vi "ReadQualisysFile.vi"(4 "sortie d'erreur":errorcluster caption="entrée d'erreur", 6 "QualisysDataType":enum16{"6DOF", "3DTracking", "6DOF + 3D"}(ring), 7 "FichierQualisys":path=path "D:/Mesures/rururu/MeasQualisys/TestValise0017.tsv") -> (0 "error out":errorcluster, 3 "QualisysWaveforms":waveform(dbl)[](graph))   [LabVIEW 2017]
uses:
  <vilib>/Utility/miscctls.llb/LVDateTimeRec.ctl
panel:
  out "NbFrames 2":u32
  out "NbCameras 2":u32
  out "NbMarkers":u32
  out "horodatage 2":timestamp=timestamp(3568107998 s since 1904-01-01)
  out "Noms des Markers":string[](array[string])
  out "Noms des colonnes 2":string[](array[string])
  out "Freq 2":u32
  out "dt 2":dbl
  out "dt":dbl
  out "Freq":u32
  out "Noms des colonnes":string[](array[string])
  out "Noms des bodies":string[](array[string])
  out "horodatage":timestamp=timestamp(3568107998 s since 1904-01-01)
  out "NbBodies":u32
  out "NbCameras":u32
  out "NbFrames":u32
  # "6DOF indicators"
  # "3D Data indicators"
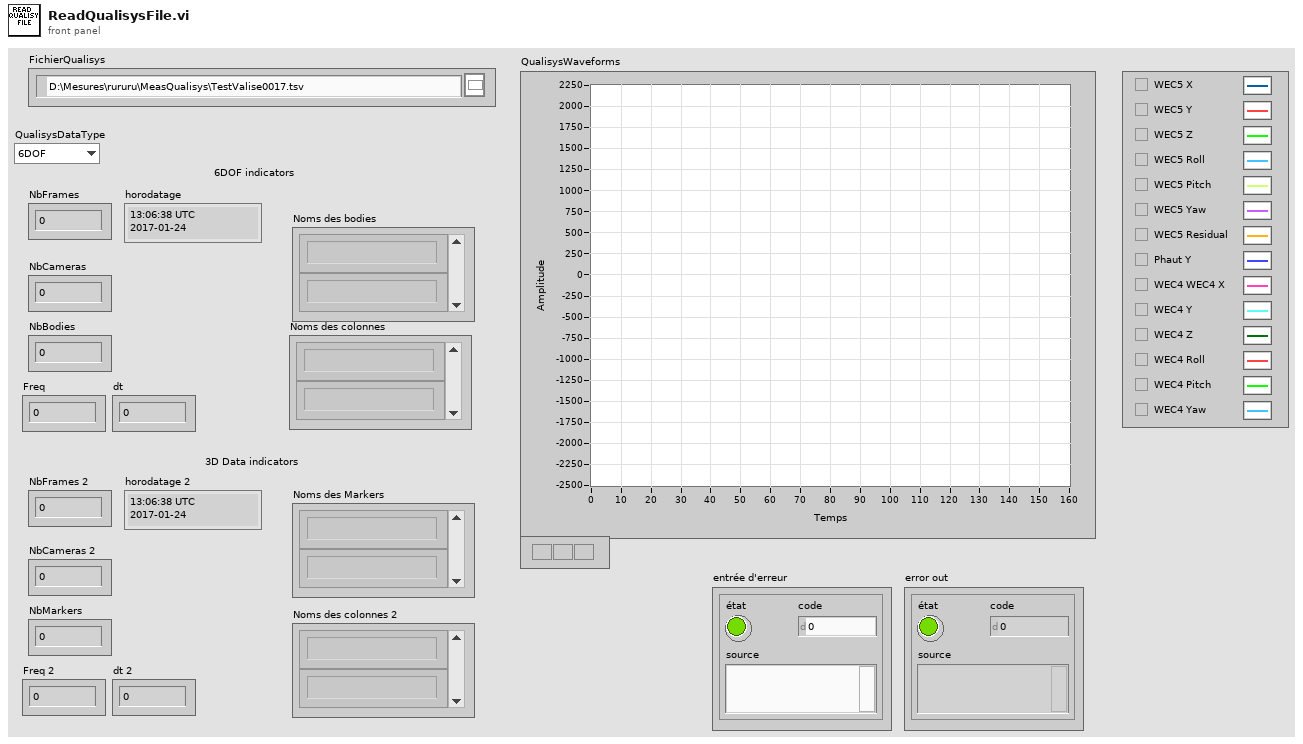
[diagram p1: front panel]
types:
  T1 = typedef "LVDateTimeRec.ctl" = cluster{"fractional second":dbl, "second":i32, "minute":i32, "hour":i32, "day of month":i32, "month":i32, "year":i32, "day of week":i32, "day of year":i32, "DST":i32}
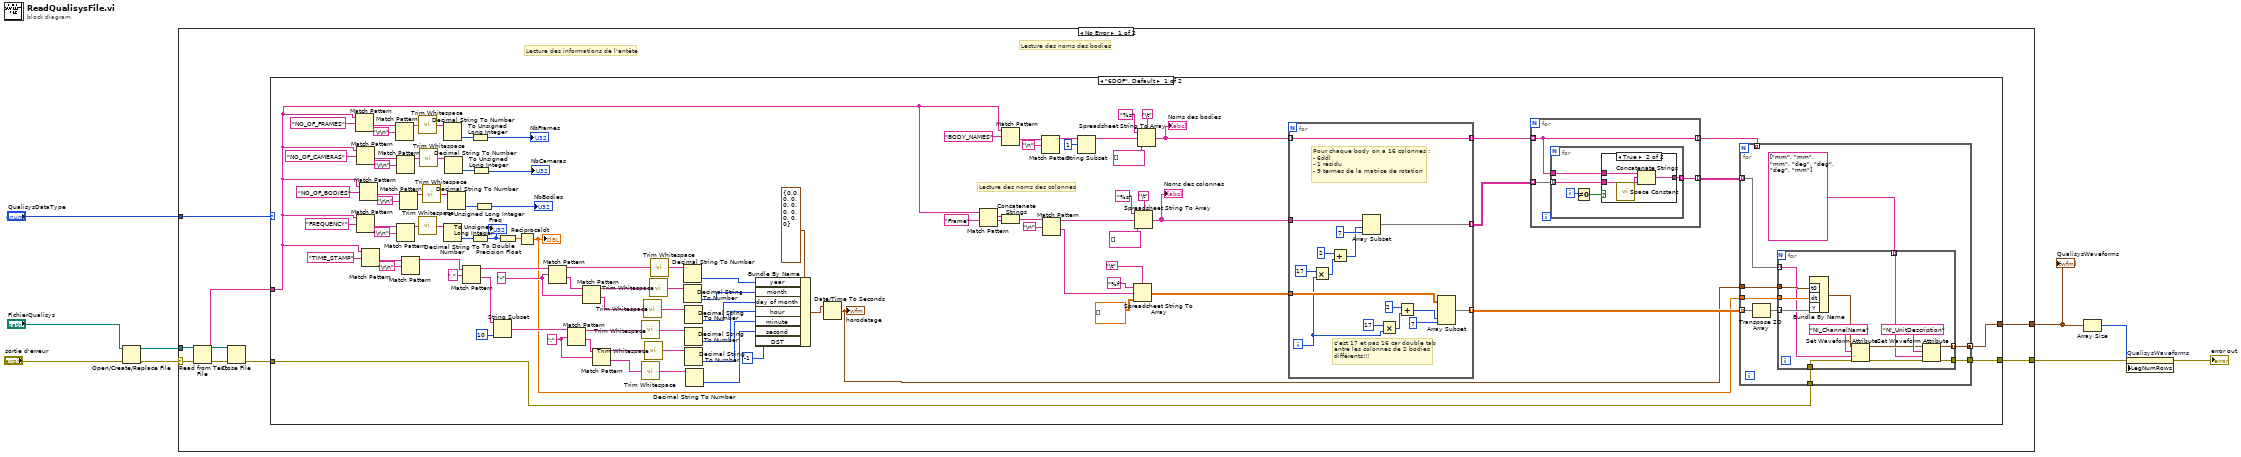
[diagram p0: block diagram]
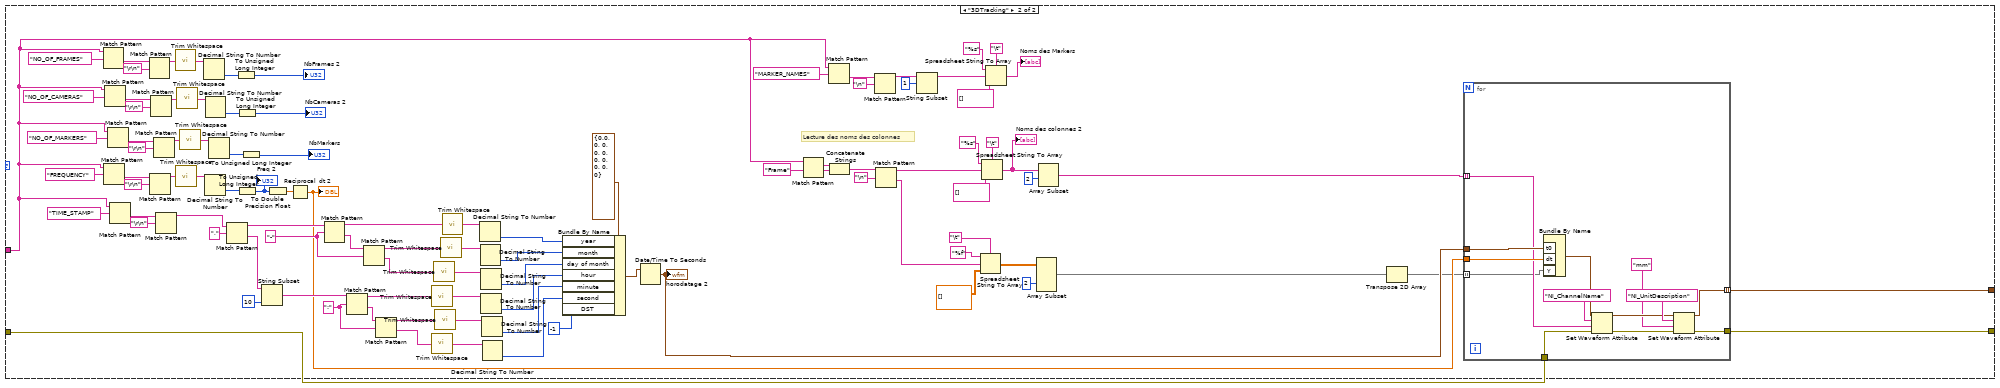
[diagram p3: hidden frame]
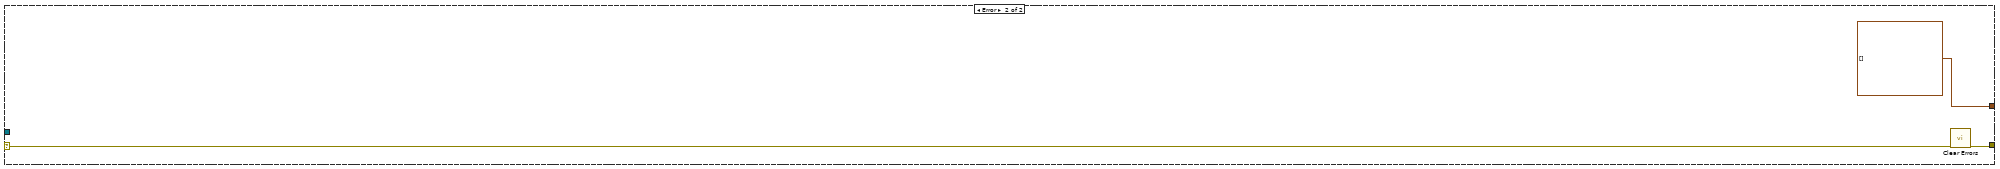
[diagram p4: hidden frame]
diagram:
  n1 = Open/Create/Replace File(file path (use dialog)="FichierQualisys", error in="sortie d'erreur") -> (refnum out=w6:refnum<file>, error out=w9:errorcluster)  [unwired: 4 in, 1 out]
  n2 = case shown="No Error" w9 {
    selector: w9 -> [w16 w281]
    tunnel: w6 -> [w15 _]
    tunnel: [w12 w282] -> w4
    tunnel: [w11 waveform(dbl)[] []] -> w5
    tunnel: "QualisysDataType" -> [w10 _]
    frame No Error {
      # "Lecture des noms des bodies"
      # "Lecture des informations de l'entête"
      n3 = Read from Text File(file (use dialog)=w15, error in=w16) -> (refnum out=w17:refnum<file>, text=w14:string, error out=w18:errorcluster)  [unwired: 2 in, 1 out]
      n4 = Close File(refnum=w17, error in=w18) -> (error out=w13:errorcluster)  [unwired: 1 out]
      n5 = case shown="\"6DOF\", Default" w10 {
        tunnel: w14 -> [w30 w185]
        tunnel: w13 -> [w22 w180]
        tunnel: [w21 w179] -> w12
        tunnel: [w20 w170] -> w11
        frame "6DOF", Default {
          w77 = ":" ("expression régulière")
          w87 = "-" ("expression régulière")
          # "Lecture des noms des colonnes"
          n6 = Match Pattern(string=w30, regular expression="NO_OF_FRAMES" ("expression régulière")) -> (after substring=w115:string)  [unwired: 1 in, 3 out]
          n7 = Match Pattern(string=w30, regular expression="FREQUENCY" ("expression régulière")) -> (after substring=w33:string)  [unwired: 1 in, 3 out]
          n8 = Match Pattern(string=w30, regular expression="NO_OF_CAMERAS" ("expression régulière")) -> (after substring=w107:string)  [unwired: 1 in, 3 out]
          n9 = Match Pattern(string=w30, regular expression="NO_OF_BODIES" ("expression régulière")) -> (after substring=w102:string)  [unwired: 1 in, 3 out]
          n10 = Match Pattern(string=w30, regular expression="TIME_STAMP" ("expression régulière")) -> (after substring=w98:string)  [unwired: 1 in, 3 out]
          n11 = Match Pattern(string=w115, regular expression="\r\n") -> (before substring=w112:string)  [unwired: 1 in, 3 out]
          n12 = Match Pattern(string=w33, regular expression="\r\n") -> (before substring=w35:string)  [unwired: 1 in, 3 out]
          n13 = Match Pattern(string=w107, regular expression="\r\n") -> (before substring=w109:string)  [unwired: 1 in, 3 out]
          n14 = Match Pattern(string=w102, regular expression="\r\n") -> (before substring=w100:string)  [unwired: 1 in, 3 out]
          n15 = Match Pattern(string=w98, regular expression="\r\n") -> (before substring=w94:string)  [unwired: 1 in, 3 out]
          n16 = call <vilib>:"Trim Whitespace.vi"("string"=w112) -> ("trimmed string"=w111:string)  [unwired: 1 in]
          n17 = call <vilib>:"Trim Whitespace.vi"("string"=w35) -> ("trimmed string"=w36:string)  [unwired: 1 in]
          n18 = call <vilib>:"Trim Whitespace.vi"("string"=w109) -> ("trimmed string"=w110:string)  [unwired: 1 in]
          n19 = call <vilib>:"Trim Whitespace.vi"("string"=w100) -> ("trimmed string"=w99:string)  [unwired: 1 in]
          n20 = Decimal String To Number(string=w111) -> (number=w114:i32)  [unwired: 2 in, 1 out]
          n21 = Decimal String To Number(string=w36) -> (number=w34:i32)  [unwired: 2 in, 1 out]
          n22 = Decimal String To Number(string=w110) -> (number=w108:i32)  [unwired: 2 in, 1 out]
          n23 = Decimal String To Number(string=w99) -> (number=w101:i32)  [unwired: 2 in, 1 out]
          n24 = Match Pattern(string=w94, regular expression="," ("expression régulière")) -> (before substring=w89:string, after substring=w75:string)  [unwired: 1 in, 2 out]
          n25 = To Unsigned Long Integer(number=w114) -> (unsigned 32bit integer=→"NbFrames":u32)
          n26 = To Unsigned Long Integer(number=w34) -> (unsigned 32bit integer=w26:u32)
          "Freq" <- w26
          n27 = To Unsigned Long Integer(number=w108) -> (unsigned 32bit integer=→"NbCameras":u32)
          n28 = To Unsigned Long Integer(number=w101) -> (unsigned 32bit integer=→"NbBodies":u32)
          n29 = String Subset(string=w75, length (rest)=10 ("longueur (reste)")) -> (substring=w74:string)  [unwired: 1 in]
          n30 = To Double Precision Float(number=w26) -> (double precision float=w25:dbl)
          n31 = Reciprocal(x=w25) -> (1/x=w24:dbl)
          "dt" <- w24
          n32 = Match Pattern(string=w89, regular expression=w87) -> (before substring=w86:string, after substring=w88:string)  [unwired: 1 in, 2 out]
          n33 = Match Pattern(string=w74, regular expression=w77) -> (before substring=w78:string, after substring=w76:string)  [unwired: 1 in, 2 out]
          n34 = Match Pattern(string=w88, regular expression=w87) -> (before substring=w84:string, after substring=w83:string)  [unwired: 1 in, 2 out]
          n35 = Match Pattern(string=w76, regular expression=w77) -> (before substring=w79:string, after substring=w80:string)  [unwired: 1 in, 2 out]
          n36 = call <vilib>:"Trim Whitespace.vi"("string"=w78) -> ("trimmed string"=w66:string)  [unwired: 1 in]
          n37 = call <vilib>:"Trim Whitespace.vi"("string"=w80) -> ("trimmed string"=w64:string)  [unwired: 1 in]
          n38 = call <vilib>:"Trim Whitespace.vi"("string"=w83) -> ("trimmed string"=w67:string)  [unwired: 1 in]
          n39 = call <vilib>:"Trim Whitespace.vi"("string"=w79) -> ("trimmed string"=w65:string)  [unwired: 1 in]
          n40 = call <vilib>:"Trim Whitespace.vi"("string"=w84) -> ("trimmed string"=w68:string)  [unwired: 1 in]
          n41 = call <vilib>:"Trim Whitespace.vi"("string"=w86) -> ("trimmed string"=w69:string)  [unwired: 1 in]
          n42 = Decimal String To Number(string=w69) -> (number=w85:i32)  [unwired: 2 in, 1 out]
          n43 = Decimal String To Number(string=w68) -> (number=w82:i32)  [unwired: 2 in, 1 out]
          n44 = Decimal String To Number(string=w67) -> (number=w81:i32)  [unwired: 2 in, 1 out]
          n45 = Decimal String To Number(string=w66) -> (number=w72:i32)  [unwired: 2 in, 1 out]
          n46 = Decimal String To Number(string=w65) -> (number=w71:i32)  [unwired: 2 in, 1 out]
          n47 = Decimal String To Number(string=w64) -> (number=w70:i32)  [unwired: 2 in, 1 out]
          n48 = Bundle By Name(cluster=T1 {"fractional second"=0.0, "second"=0, "minute"=0, "hour"=0, "day of month"=0, "month"=0, "year"=0, "day of week"=0, "day of year"=0, "DST"=0} ("cluster date/heure"), "year"=w85, "month"=w82, "day of month"=w81, "hour"=w72, "minute"=w71, "second"=w70, "DST"=-1) -> (w92:T1)
          n49 = Date/Time To Seconds(2:w92) -> (0:w23:timestamp)  [unwired: 1 in]
          "horodatage" <- w23
          n50 = Match Pattern(string=w30, regular expression="Frame" ("expression régulière")) -> (match substring=w49:string, after substring=w48:string)  [unwired: 1 in, 2 out]
          n51 = Match Pattern(string=w30, regular expression="BODY_NAMES" ("expression régulière")) -> (after substring=w63:string)  [unwired: 1 in, 3 out]
          n52 = Concatenate Strings(w49, w48) -> (w47:string)
          n53 = Match Pattern(string=w63, regular expression="\n") -> (before substring=w60:string)  [unwired: 1 in, 3 out]
          n54 = Match Pattern(string=w47, regular expression="\n") -> (before substring=w46:string, after substring=w45:string)  [unwired: 1 in, 2 out]
          n55 = String Subset(string=w60, offset (0)=1) -> (substring=w56:string)  [unwired: 1 in]
          n56 = Spreadsheet String To Array(delimiter (Tab)="\t", format string="%f" ("chaîne de format"), spreadsheet string=w45, array type (2D Dbl)=dbl[][] [] ("type de tableau (2D de dbl)")) -> (array=w39:dbl[][])
          n57 = Spreadsheet String To Array(delimiter (Tab)="\t", format string="%s" ("chaîne de format"), spreadsheet string=w46, array type (2D Dbl)=string[] [] ("type de tableau (2D de dbl)")) -> (array=w40:string[])
          "Noms des colonnes" <- w40
          n58 = Spreadsheet String To Array(delimiter (Tab)="\t", format string="%s" ("chaîne de format"), spreadsheet string=w56, array type (2D Dbl)=string[] [] ("type de tableau (2D de dbl)")) -> (array=w41:string[])
          "Noms des bodies" <- w41
          n59 = for {
            tunnel: w40 -> [w158]
            tunnel: w41 -> [w153] mode=indexing
            tunnel: [w157] -> w38 mode=indexing
            tunnel: w39 -> [w156]
            tunnel: [w154] -> w27 mode=indexing
            tunnel: [w153] -> w37 mode=indexing
            i -> [w155]
            # "Pour chaque body on a 16 colonnes :\n- 6ddl\n- 1 résidu\n- 9 termes de la matrice de rotation"
            # "c'est 17 et pas 16 car double tab\nentre les colonnes de 2 bodies\ndifférents!!!"
            n60 = Multiply(x=17 ("indice"), y=w155) -> (x*y=w166:i32)
            n61 = Add(x=2 ("indice"), y=w166) -> (x+y=w163:i32)
            n62 = Array Subset(array=w158, index=w163, length=7 ("longueur")) -> (w157:string[])
            n63 = Multiply(x=17 ("indice"), y=w155) -> (x*y=w160:i32)
            n64 = Add(x=2 ("indice"), y=w160) -> (x+y=w159:i32)
            n65 = Array Subset(array=w156, index (col)=w159, length (col)=7 ("longueur")) -> (w154:dbl[][])  [unwired: 2 in]
          }
          n66 = for {
            tunnel: w38 -> [w142] mode=indexing
            tunnel: [w141] -> w28 mode=indexing
            tunnel: w37 -> [w140] mode=indexing
            tunnel: [w140] -> w29 mode=indexing
            n67 = for {
              tunnel: w142 -> [w147] mode=indexing
              tunnel: [w146] -> w141 mode=indexing
              tunnel: w140 -> [w143]
              i -> [w145]
              n68 = Not Equal To 0?(x=w145) -> (x != 0?=w144:bool)
              n69 = case shown="True" w144 {
                tunnel: w147 -> [w148 w151]
                tunnel: [w148 w152] -> w146
                tunnel: w143 -> [_ w149]
                frame False {
                }
                frame True {
                  n70 = call <vilib>:"Space Constant.vi"() -> ("String"=w150:string)
                  n71 = Concatenate Strings(w149, w150, w151) -> (w152:string)
                }
              }
            }
          }
          n72 = for {
            tunnel: w29 -> [_] mode=indexing
            tunnel: w28 -> [w120] mode=indexing
            tunnel: w27 -> [w124] mode=indexing
            tunnel: w24 -> [w125]
            tunnel: w23 -> [w126]
            tunnel: w22 -> [w122]
            tunnel: [w121] -> w21
            tunnel: [w118] -> w20 mode=concatenating
            n73 = Transpose 2D Array(2D array=w124) -> (transposed array=w123:dbl[][])
            n74 = for {
              tunnel: w126 -> [w139]
              tunnel: w125 -> [w138]
              tunnel: w123 -> [w137] mode=indexing
              tunnel: w122 -> [w131]
              tunnel: [w130] -> w121
              tunnel: w120 -> [w129] mode=indexing
              tunnel: string[] ["mm", "mm", "mm", "deg", "deg", "deg", "mm"] -> [w128] mode=indexing
              tunnel: [w127] -> w118 mode=indexing
              n75 = Bundle By Name("t0"=w139, "dt"=w138, "Y"=w137) -> (w132:waveform(dbl))  [unwired: 1 in]
              n76 = Set Waveform Attribute(4:w131, 5:w129, 6:"NI_ChannelName" ("nom"), 7:w132) -> (0:w134:errorcluster, 3:w133:waveform(dbl))  [unwired: 1 out]
              n77 = Set Waveform Attribute(4:w134, 5:w128, 6:"NI_UnitDescription" ("nom"), 7:w133) -> (0:w130:errorcluster, 3:w127:waveform(dbl))  [unwired: 1 out]
            }
          }
        }
        frame "3DTracking" {
          w227 = ":" ("expression régulière")
          w237 = "-" ("expression régulière")
          # "Lecture des noms des colonnes"
          n78 = Match Pattern(string=w185, regular expression="NO_OF_FRAMES" ("expression régulière")) -> (after substring=w265:string)  [unwired: 1 in, 3 out]
          n79 = Match Pattern(string=w185, regular expression="FREQUENCY" ("expression régulière")) -> (after substring=w188:string)  [unwired: 1 in, 3 out]
          n80 = Match Pattern(string=w185, regular expression="NO_OF_CAMERAS" ("expression régulière")) -> (after substring=w257:string)  [unwired: 1 in, 3 out]
          n81 = Match Pattern(string=w185, regular expression="NO_OF_MARKERS" ("expression régulière")) -> (after substring=w252:string)  [unwired: 1 in, 3 out]
          n82 = Match Pattern(string=w185, regular expression="TIME_STAMP" ("expression régulière")) -> (after substring=w248:string)  [unwired: 1 in, 3 out]
          n83 = Match Pattern(string=w265, regular expression="\r\n") -> (before substring=w262:string)  [unwired: 1 in, 3 out]
          n84 = Match Pattern(string=w188, regular expression="\r\n") -> (before substring=w190:string)  [unwired: 1 in, 3 out]
          n85 = Match Pattern(string=w257, regular expression="\r\n") -> (before substring=w259:string)  [unwired: 1 in, 3 out]
          n86 = Match Pattern(string=w252, regular expression="\r\n") -> (before substring=w250:string)  [unwired: 1 in, 3 out]
          n87 = Match Pattern(string=w248, regular expression="\r\n") -> (before substring=w244:string)  [unwired: 1 in, 3 out]
          n88 = call <vilib>:"Trim Whitespace.vi"("string"=w262) -> ("trimmed string"=w261:string)  [unwired: 1 in]
          n89 = call <vilib>:"Trim Whitespace.vi"("string"=w190) -> ("trimmed string"=w191:string)  [unwired: 1 in]
          n90 = call <vilib>:"Trim Whitespace.vi"("string"=w259) -> ("trimmed string"=w260:string)  [unwired: 1 in]
          n91 = call <vilib>:"Trim Whitespace.vi"("string"=w250) -> ("trimmed string"=w249:string)  [unwired: 1 in]
          n92 = Decimal String To Number(string=w261) -> (number=w264:i32)  [unwired: 2 in, 1 out]
          n93 = Decimal String To Number(string=w191) -> (number=w189:i32)  [unwired: 2 in, 1 out]
          n94 = Decimal String To Number(string=w260) -> (number=w258:i32)  [unwired: 2 in, 1 out]
          n95 = Decimal String To Number(string=w249) -> (number=w251:i32)  [unwired: 2 in, 1 out]
          n96 = Match Pattern(string=w244, regular expression="," ("expression régulière")) -> (before substring=w239:string, after substring=w225:string)  [unwired: 1 in, 2 out]
          n97 = To Unsigned Long Integer(number=w264) -> (unsigned 32bit integer=→"NbFrames 2":u32)
          n98 = To Unsigned Long Integer(number=w189) -> (unsigned 32bit integer=w184:u32)
          "Freq 2" <- w184
          n99 = To Unsigned Long Integer(number=w258) -> (unsigned 32bit integer=→"NbCameras 2":u32)
          n100 = To Unsigned Long Integer(number=w251) -> (unsigned 32bit integer=→"NbMarkers":u32)
          n101 = String Subset(string=w225, length (rest)=10 ("longueur (reste)")) -> (substring=w224:string)  [unwired: 1 in]
          n102 = To Double Precision Float(number=w184) -> (double precision float=w183:dbl)
          n103 = Reciprocal(x=w183) -> (1/x=w182:dbl)
          "dt 2" <- w182
          n104 = Match Pattern(string=w239, regular expression=w237) -> (before substring=w236:string, after substring=w238:string)  [unwired: 1 in, 2 out]
          n105 = Match Pattern(string=w224, regular expression=w227) -> (before substring=w228:string, after substring=w226:string)  [unwired: 1 in, 2 out]
          n106 = Match Pattern(string=w238, regular expression=w237) -> (before substring=w234:string, after substring=w233:string)  [unwired: 1 in, 2 out]
          n107 = Match Pattern(string=w226, regular expression=w227) -> (before substring=w229:string, after substring=w230:string)  [unwired: 1 in, 2 out]
          n108 = call <vilib>:"Trim Whitespace.vi"("string"=w228) -> ("trimmed string"=w216:string)  [unwired: 1 in]
          n109 = call <vilib>:"Trim Whitespace.vi"("string"=w230) -> ("trimmed string"=w214:string)  [unwired: 1 in]
          n110 = call <vilib>:"Trim Whitespace.vi"("string"=w233) -> ("trimmed string"=w217:string)  [unwired: 1 in]
          n111 = call <vilib>:"Trim Whitespace.vi"("string"=w229) -> ("trimmed string"=w215:string)  [unwired: 1 in]
          n112 = call <vilib>:"Trim Whitespace.vi"("string"=w234) -> ("trimmed string"=w218:string)  [unwired: 1 in]
          n113 = call <vilib>:"Trim Whitespace.vi"("string"=w236) -> ("trimmed string"=w219:string)  [unwired: 1 in]
          n114 = Decimal String To Number(string=w219) -> (number=w235:i32)  [unwired: 2 in, 1 out]
          n115 = Decimal String To Number(string=w218) -> (number=w232:i32)  [unwired: 2 in, 1 out]
          n116 = Decimal String To Number(string=w217) -> (number=w231:i32)  [unwired: 2 in, 1 out]
          n117 = Decimal String To Number(string=w216) -> (number=w222:i32)  [unwired: 2 in, 1 out]
          n118 = Decimal String To Number(string=w215) -> (number=w221:i32)  [unwired: 2 in, 1 out]
          n119 = Decimal String To Number(string=w214) -> (number=w220:i32)  [unwired: 2 in, 1 out]
          n120 = Bundle By Name(cluster=T1 {"fractional second"=0.0, "second"=0, "minute"=0, "hour"=0, "day of month"=0, "month"=0, "year"=0, "day of week"=0, "day of year"=0, "DST"=0} ("cluster date/heure"), "year"=w235, "month"=w232, "day of month"=w231, "hour"=w222, "minute"=w221, "second"=w220, "DST"=-1) -> (w242:T1)
          n121 = Date/Time To Seconds(2:w242) -> (0:w181:timestamp)  [unwired: 1 in]
          "horodatage 2" <- w181
          n122 = Match Pattern(string=w185, regular expression="Frame" ("expression régulière")) -> (match substring=w199:string, after substring=w198:string)  [unwired: 1 in, 2 out]
          n123 = Match Pattern(string=w185, regular expression="MARKER_NAMES" ("expression régulière")) -> (after substring=w213:string)  [unwired: 1 in, 3 out]
          n124 = Concatenate Strings(w199, w198) -> (w197:string)
          n125 = Match Pattern(string=w213, regular expression="\n") -> (before substring=w210:string)  [unwired: 1 in, 3 out]
          n126 = Match Pattern(string=w197, regular expression="\n") -> (before substring=w196:string, after substring=w195:string)  [unwired: 1 in, 2 out]
          n127 = String Subset(string=w210, offset (0)=1) -> (substring=w206:string)  [unwired: 1 in]
          n128 = Spreadsheet String To Array(delimiter (Tab)="\t", format string="%f" ("chaîne de format"), spreadsheet string=w195, array type (2D Dbl)=dbl[][] [] ("type de tableau (2D de dbl)")) -> (array=w177:dbl[][])
          n129 = Spreadsheet String To Array(delimiter (Tab)="\t", format string="%s" ("chaîne de format"), spreadsheet string=w196, array type (2D Dbl)=string[] [] ("type de tableau (2D de dbl)")) -> (array=w175:string[])
          "Noms des colonnes 2" <- w175
          n130 = Spreadsheet String To Array(delimiter (Tab)="\t", format string="%s" ("chaîne de format"), spreadsheet string=w206, array type (2D Dbl)=string[] [] ("type de tableau (2D de dbl)")) -> (array=→"Noms des Markers":string[])
          n131 = Array Subset(array=w177, index (col)=2 ("index")) -> (w172:dbl[][])  [unwired: 3 in]
          n132 = Array Subset(array=w175, index=2) -> (w171:string[])  [unwired: 1 in]
          n133 = Transpose 2D Array(2D array=w172) -> (transposed array=w169:dbl[][])
          n134 = for {
            tunnel: w169 -> [w268] mode=indexing
            tunnel: w182 -> [w279]
            tunnel: w181 -> [w280]
            tunnel: w180 -> [w278]
            tunnel: [w277] -> w179
            tunnel: w171 -> [w270] mode=indexing
            tunnel: [w269] -> w170 mode=indexing
            n135 = Bundle By Name("t0"=w280, "dt"=w279, "Y"=w268) -> (w272:waveform(dbl))  [unwired: 1 in]
            n136 = Set Waveform Attribute(4:w278, 5:w270, 6:"NI_ChannelName" ("nom"), 7:w272) -> (0:w274:errorcluster, 3:w273:waveform(dbl))  [unwired: 1 out]
            n137 = Set Waveform Attribute(4:w274, 5:"mm" ("expression régulière"), 6:"NI_UnitDescription" ("nom"), 7:w273) -> (0:w277:errorcluster, 3:w269:waveform(dbl))  [unwired: 1 out]
          }
        }
      }
    }
    frame Error {
      n138 = call <vilib>:"Clear Errors.vi"("error in (no error)"=w281) -> ("error out"=w282:errorcluster)  [unwired: 5 in, 1 out]
    }
  }
  "QualisysWaveforms" <- w5
  n139 = Array Size(array=w5) -> (size(s)=w2:i32)
  n140 = property on="QualisysWaveforms" class="WFGraph (strict)"(error in=w4, "LegNumRows"=w2) -> (error out=→"error out":errorcluster)  [unwired: 1 in, 1 out]
